vi "keyboard_mouse_stuff.vi"() -> ()   [LabVIEW 2011]
uses:
  <vilib>/Utility/inputDevices.llb/closeMouse.vi
  <vilib>/Utility/inputDevices.llb/closeKeyboard.vi
  <vilib>/Utility/inputDevices.llb/mouseAcquire.vi
  <vilib>/Utility/inputDevices.llb/keyboardAcquire.vi
panel:
  out "button 2":bool
  out "button 1":bool
  out "Scrolling":i32
  out "Vertical":i32
  out "Horizontal":i32
  in  "error in (no error)":errorcluster
  out "error out 2":errorcluster
  out "RIGHT":bool
  out "DOWN":bool
  out "LEFT":bool
  out "UP":bool
  in  "stop":bool
  out "keys pressed":T1(array[ring])
  out "error out":errorcluster
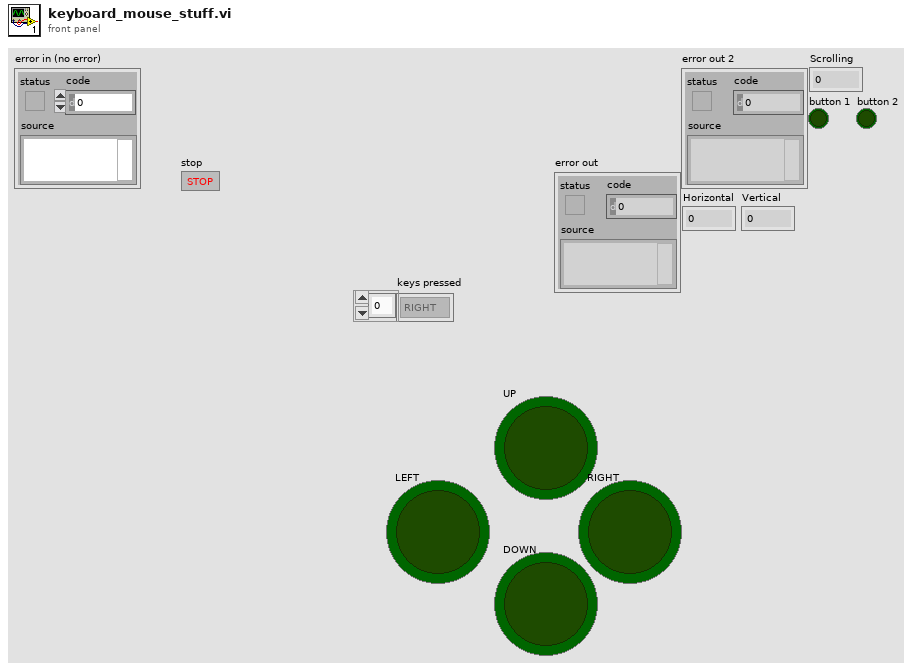
[diagram p1: front panel]
types:
  T1 = enum16{"0", "1", "2", "3", "4", "5", "6", "7", "8", "9", "A", "B", "C", "D", "E", "F", "G", "H", "I", "J", "K", "L", "M", "N", "O", "P", "Q", "R", "S", "T", "U", "V", "W", "X", "Y", "Z", "F1", "F2", "F3", "F4", "F5", "F6", "F7", "F8", "F9", "F10", "F11", "F12", "F13", "F14", "F15", "ADD", "BACK", "BACKSLASH", "CAPITAL", "COMMA", "DECIMAL", "DELETE", "DIVIDE", "DOWN", "END", "EQUALS", "ESCAPE", "GRAVE (`)", "HOME", "INSERT", "LBRACKET", "LCONTROL", "LEFT", "L ALT", "LSHIFT", "LWIN", "MINUS", "MULTIPLY", "NEXT", "NUMLOCK", "NUMPAD_0", "NUMPAD_1", "NUMPAD_2", "NUMPAD_3", "NUMPAD_4", "NUMPAD_5", "NUMPAD_6", "NUMPAD_7", "NUMPAD_8", "NUMPAD_9", "PAUSE", "PERIOD", "PRIOR (PG UP)", "RBRACKET", "RCONTROL", "RETURN", "RIGHT", "R ALT", "RSHIFT", "RWIN", "SCROLL", "SEMICOLON", "SLASH", "SPACE", "SUBTRACT", "TAB", "UP", "ENTER (num pad)", "' (quote)"}[]
  T2 = cluster{"Horizontal":i32, "Vertical":i32, "Scrolling":i32}
  T3 = cluster{"button 1":bool, "button 2":bool, "button 3":bool, "button 4":bool}
  T4 = cluster{"[0]":bool, "[1]":bool, "[2]":bool, "[3]":bool, "[4]":bool, "[5]":bool, "[6]":bool, "[7]":bool, "[8]":bool}
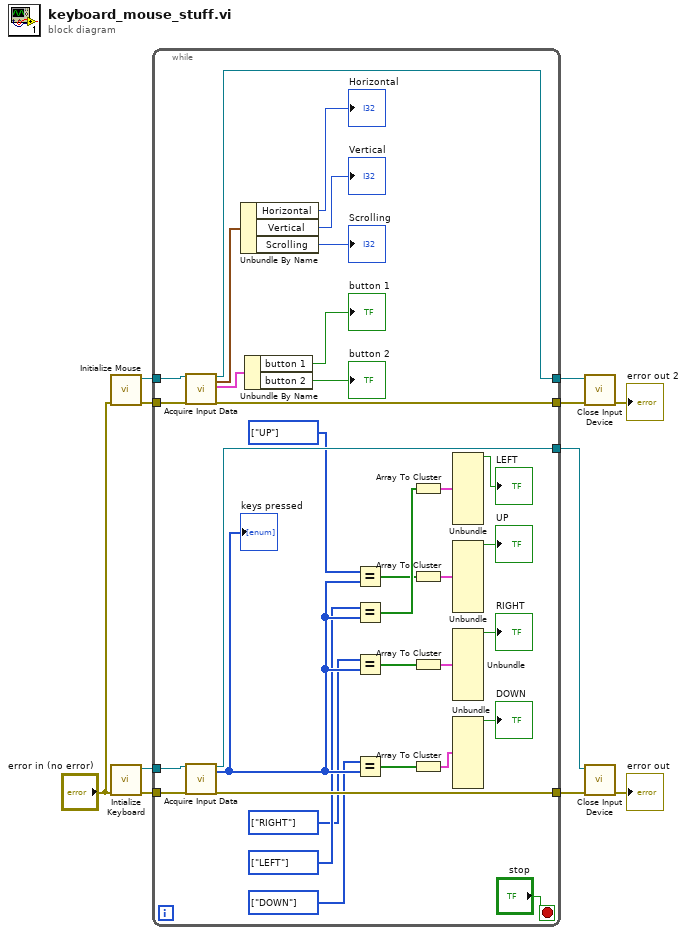
[diagram p0: block diagram]
diagram:
  n1 = call <vilib>:"Initialize Mouse.vi"("error in (no error)"="error in (no error)") -> ("error out"=w5:errorcluster, "device ID"=w6:refnum<k1>)  [unwired: 9 in]
  n2 = call <vilib>:"Intialize Keyboard.vi"("error in (no error)"="error in (no error)") -> ("error out"=w10:errorcluster, "device ID"=w11:refnum<k1>)  [unwired: 9 in]
  n3 = while {
    tunnel: w11 -> [w44]
    tunnel: w10 -> [w43]
    tunnel: [w42] -> w9
    tunnel: [w41] -> w8
    tunnel: w6 -> [w22]
    tunnel: w5 -> [w21]
    tunnel: [w20] -> w4
    tunnel: [w19] -> w3
    stop <- "stop" stop-if-true
    w35 = T1 [enum."RIGHT"] items=["0", "1", "2", "3", "4", "5", "6", "7", "8", "9", "A", "B", "C", "D", "E", "F", "G", "H", "I", "J", "K", "L", "M", "N", "O", "P", "Q", "R", "S", "T", "U", "V", "W", "X", "Y", "Z", "F1", "F2", "F3", "F4", "F5", "F6", "F7", "F8", "F9", "F10", "F11", "F12", "F13", "F14", "F15", "ADD", "BACK", "BACKSLASH", "CAPITAL", "COMMA", "DECIMAL", "DELETE", "DIVIDE", "DOWN", "END", "EQUALS", "ESCAPE", "GRAVE (`)", "HOME", "INSERT", "LBRACKET", "LCONTROL", "LEFT", "L ALT", "LSHIFT", "LWIN", "MINUS", "MULTIPLY", "NEXT", "NUMLOCK", "NUMPAD_0", "NUMPAD_1", "NUMPAD_2", "NUMPAD_3", "NUMPAD_4", "NUMPAD_5", "NUMPAD_6", "NUMPAD_7", "NUMPAD_8", "NUMPAD_9", "PAUSE", "PERIOD", "PRIOR (PG UP)", "RBRACKET", "RCONTROL", "RETURN", "RIGHT", "R ALT", "RSHIFT", "RWIN", "SCROLL", "SEMICOLON", "SLASH", "SPACE", "SUBTRACT", "TAB", "UP", "ENTER (num pad)", "' (quote)"] ("x")
    w36 = T1 [enum."LEFT"] items=["0", "1", "2", "3", "4", "5", "6", "7", "8", "9", "A", "B", "C", "D", "E", "F", "G", "H", "I", "J", "K", "L", "M", "N", "O", "P", "Q", "R", "S", "T", "U", "V", "W", "X", "Y", "Z", "F1", "F2", "F3", "F4", "F5", "F6", "F7", "F8", "F9", "F10", "F11", "F12", "F13", "F14", "F15", "ADD", "BACK", "BACKSLASH", "CAPITAL", "COMMA", "DECIMAL", "DELETE", "DIVIDE", "DOWN", "END", "EQUALS", "ESCAPE", "GRAVE (`)", "HOME", "INSERT", "LBRACKET", "LCONTROL", "LEFT", "L ALT", "LSHIFT", "LWIN", "MINUS", "MULTIPLY", "NEXT", "NUMLOCK", "NUMPAD_0", "NUMPAD_1", "NUMPAD_2", "NUMPAD_3", "NUMPAD_4", "NUMPAD_5", "NUMPAD_6", "NUMPAD_7", "NUMPAD_8", "NUMPAD_9", "PAUSE", "PERIOD", "PRIOR (PG UP)", "RBRACKET", "RCONTROL", "RETURN", "RIGHT", "R ALT", "RSHIFT", "RWIN", "SCROLL", "SEMICOLON", "SLASH", "SPACE", "SUBTRACT", "TAB", "UP", "ENTER (num pad)", "' (quote)"] ("x")
    w37 = T1 [enum."DOWN"] items=["0", "1", "2", "3", "4", "5", "6", "7", "8", "9", "A", "B", "C", "D", "E", "F", "G", "H", "I", "J", "K", "L", "M", "N", "O", "P", "Q", "R", "S", "T", "U", "V", "W", "X", "Y", "Z", "F1", "F2", "F3", "F4", "F5", "F6", "F7", "F8", "F9", "F10", "F11", "F12", "F13", "F14", "F15", "ADD", "BACK", "BACKSLASH", "CAPITAL", "COMMA", "DECIMAL", "DELETE", "DIVIDE", "DOWN", "END", "EQUALS", "ESCAPE", "GRAVE (`)", "HOME", "INSERT", "LBRACKET", "LCONTROL", "LEFT", "L ALT", "LSHIFT", "LWIN", "MINUS", "MULTIPLY", "NEXT", "NUMLOCK", "NUMPAD_0", "NUMPAD_1", "NUMPAD_2", "NUMPAD_3", "NUMPAD_4", "NUMPAD_5", "NUMPAD_6", "NUMPAD_7", "NUMPAD_8", "NUMPAD_9", "PAUSE", "PERIOD", "PRIOR (PG UP)", "RBRACKET", "RCONTROL", "RETURN", "RIGHT", "R ALT", "RSHIFT", "RWIN", "SCROLL", "SEMICOLON", "SLASH", "SPACE", "SUBTRACT", "TAB", "UP", "ENTER (num pad)", "' (quote)"] ("x")
    w38 = T1 [enum."UP"] items=["0", "1", "2", "3", "4", "5", "6", "7", "8", "9", "A", "B", "C", "D", "E", "F", "G", "H", "I", "J", "K", "L", "M", "N", "O", "P", "Q", "R", "S", "T", "U", "V", "W", "X", "Y", "Z", "F1", "F2", "F3", "F4", "F5", "F6", "F7", "F8", "F9", "F10", "F11", "F12", "F13", "F14", "F15", "ADD", "BACK", "BACKSLASH", "CAPITAL", "COMMA", "DECIMAL", "DELETE", "DIVIDE", "DOWN", "END", "EQUALS", "ESCAPE", "GRAVE (`)", "HOME", "INSERT", "LBRACKET", "LCONTROL", "LEFT", "L ALT", "LSHIFT", "LWIN", "MINUS", "MULTIPLY", "NEXT", "NUMLOCK", "NUMPAD_0", "NUMPAD_1", "NUMPAD_2", "NUMPAD_3", "NUMPAD_4", "NUMPAD_5", "NUMPAD_6", "NUMPAD_7", "NUMPAD_8", "NUMPAD_9", "PAUSE", "PERIOD", "PRIOR (PG UP)", "RBRACKET", "RCONTROL", "RETURN", "RIGHT", "R ALT", "RSHIFT", "RWIN", "SCROLL", "SEMICOLON", "SLASH", "SPACE", "SUBTRACT", "TAB", "UP", "ENTER (num pad)", "' (quote)"] ("x")
    n4 = call-poly <vilib>:"Acquire Input Data.vi"("device ID"=w22, "error in (no error)"=w21) -> ("device ID"=w20:refnum<k1>, "axis info"=w18:T2, "button info"=w14:T3, "error out"=w19:errorcluster)  [unwired: 14 in]
    n5 = call-poly <vilib>:"Acquire Input Data.vi"("device ID"=w44, "error in (no error)"=w43) -> ("device ID"=w41:refnum<k1>, "keys pressed"=w39:T1, "error out"=w42:errorcluster)  [unwired: 15 in]
    "keys pressed" <- w39
    n6 = Unbundle By Name(w18) -> ("Horizontal"=→"Horizontal":i32, "Vertical"=→"Vertical":i32, "Scrolling"=→"Scrolling":i32)
    n7 = Unbundle By Name(w14) -> ("button 1"=→"button 1":bool, "button 2"=→"button 2":bool)
    n8 = Equal?(x=w38, y=w39) -> (x = y?=w24:bool[])
    n9 = Equal?(x=w36, y=w39) -> (x = y?=w30:bool[])
    n10 = Equal?(x=w35, y=w39) -> (x = y?=w34:bool[])
    n11 = Equal?(x=w37, y=w39) -> (x = y?=w27:bool[])
    n12 = Array To Cluster(array=w30) -> (cluster=w31:T4)
    n13 = Array To Cluster(array=w24) -> (cluster=w25:T4)
    n14 = Array To Cluster(array=w34) -> (cluster=w33:T4)
    n15 = Array To Cluster(array=w27) -> (cluster=w28:T4)
    n16 = Unbundle(w31) -> ("[0]"=→"LEFT":bool)  [unwired: 8 out]
    n17 = Unbundle(w25) -> ("[0]"=→"UP":bool)  [unwired: 8 out]
    n18 = Unbundle(w33) -> ("[0]"=→"RIGHT":bool)  [unwired: 8 out]
    n19 = Unbundle(w28) -> ("[0]"=→"DOWN":bool)  [unwired: 8 out]
  }
  n20 = call-poly <vilib>:"Close Input Device.vi"("error in (no error)"=w3, "device ID"=w4) -> ("error out"=→"error out 2":errorcluster)  [unwired: 8 in]
  n21 = call-poly <vilib>:"Close Input Device.vi"("error in (no error)"=w9, "device ID"=w8) -> ("error out"=→"error out":errorcluster)  [unwired: 8 in]
